vi "_Is Server Running.vi"(4 "error in":errorcluster, 7 "IsSimplicityServer":bool) -> (0 "error out":errorcluster, 3 "Server Reference":refnum<vi>)   [LabVIEW 2012]
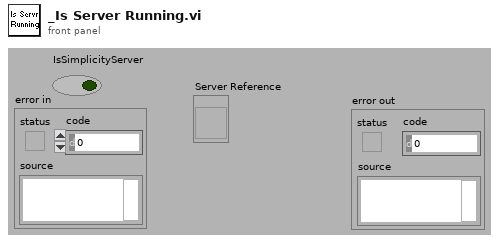
[diagram p1: front panel]
types:
  T1 = enum32{"Bad", "Idle", "Run top level", "Running"}
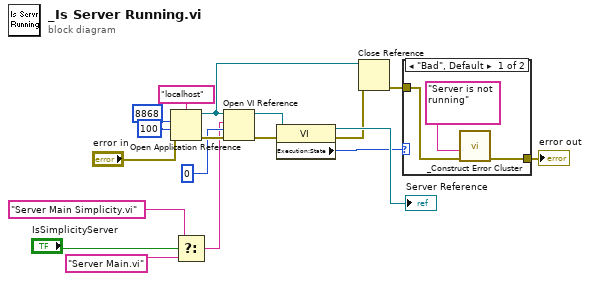
[diagram p0: block diagram]
diagram:
  n1 = Open Application Reference(8:"error in", 9:100 ("timeout ms (60000)"), 10:u32 8868 ("port number (3363)"), 11:"localhost" ("machine name (\"\":  open local reference)")) -> (0:w16:errorcluster, 3:w12:refnum<vi>)
  n2 = Select(t="Server Main Simplicity.vi" ("VI Name"), s="IsSimplicityServer", f="Server Main.vi" ("VI Name")) -> (s? t:f=w1:string)
  n3 = Open VI Reference(application reference (local)=w12, vi path=w1, options=0, error in (no error)=w16) -> (vi reference=w11:refnum<vi>, error out=w13:errorcluster)  [unwired: 2 out]
  n4 = property class="VI"(reference=w11, error in=w13) -> (reference out=→"Server Reference":refnum<vi>, error out=w9:errorcluster, "Execution:State"=w6:T1)
  n5 = Close Reference(reference=w12, error in (no error)=w9) -> (error out=w8:errorcluster)
  n6 = case shown="\"Bad\", Default" w6 {
    tunnel: w8 -> [w21 _]
    tunnel: [w19 _] -> w7
    frame "Bad", Default {
      n7 = call "_Construct Error Cluster.vi"("error in"=w21, "reason"="Server is not running") -> ("error out"=w19:errorcluster)  [unwired: 2 in, 3 out]
    }
    frame "Run top level", "Running" {
    }
  }
  "error out" <- w7
